vi "Tag Example.vi"() -> ()   [LabVIEW 2016]
uses:
  <vilib>/TagLibrary/Create Tag (Int).vi
  <vilib>/TagLibrary/Write (Int).vi
  <vilib>/TagLibrary/Close Tag (Single).vi
  <vilib>/TagLibrary/TagLibrary.lvlib
panel:
  out "error out":errorcluster
  in  "int":i32 caption="integer"
  in  "tag path":string="foo.bar"
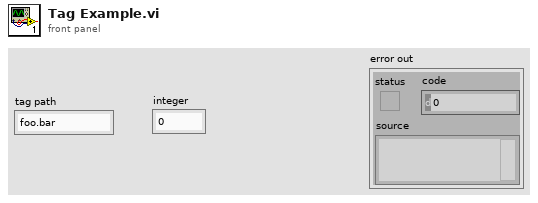
[diagram p1: front panel]
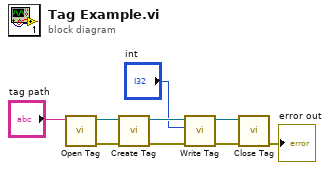
[diagram p0: block diagram]
diagram:
  n1 = call <vilib>:"Open Tag.vi"("tag path"="tag path") -> ("error out"=w2:errorcluster, "tag reference out"=w3:refnum<k21>)  [unwired: 9 in]
  n2 = call-poly <vilib>:"Create Tag.vi"("error in (no error)"=w2, "tag reference in"=w3) -> ("error out"=w5:errorcluster, "tag reference out"=w6:refnum<k21>)  [unwired: 8 in]
  n3 = call-poly <vilib>:"Write Tag.vi"("error in (no error)"=w5, "int"="int", "tag reference in"=w6) -> ("error out"=w8:errorcluster, "tag reference out"=w7:refnum<k21>)  [unwired: 7 in]
  n4 = call-poly <vilib>:"Close Tag.vi"("error in (no error)"=w8, "tag reference"=w7) -> ("error out"=→"error out":errorcluster)  [unwired: 9 in]
